vi "Control Loop Process.vi"(8 "error in (no error)":errorcluster, 9 "MainDirectionIn":string, 11 "MPC_Laser Marked in":refnum<class "MPC_Laser Marked.lvclass">) -> (0 "error out":errorcluster, 1 "MainDirectionOut":string, 2 "ProcessAction":string[](array[string]), 3 "MPC_Laser Marked out":refnum<class "MPC_Laser Marked.lvclass">)   [LabVIEW 2019, in "MPC_Laser Marked.lvclass"]
uses:
  MPC_Laser Marked.lvclass
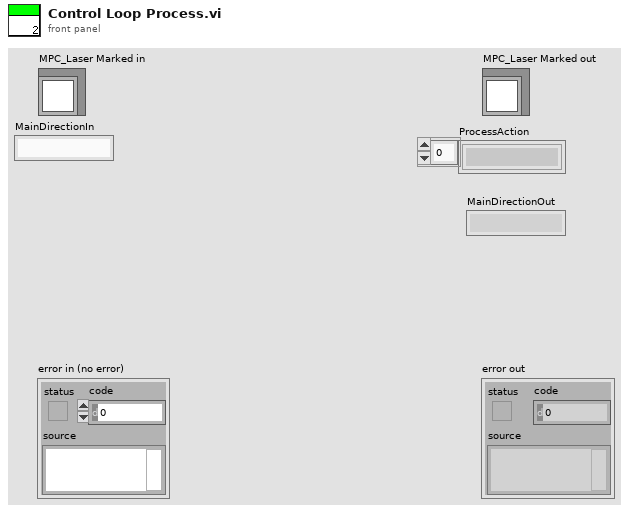
[diagram p1: front panel]
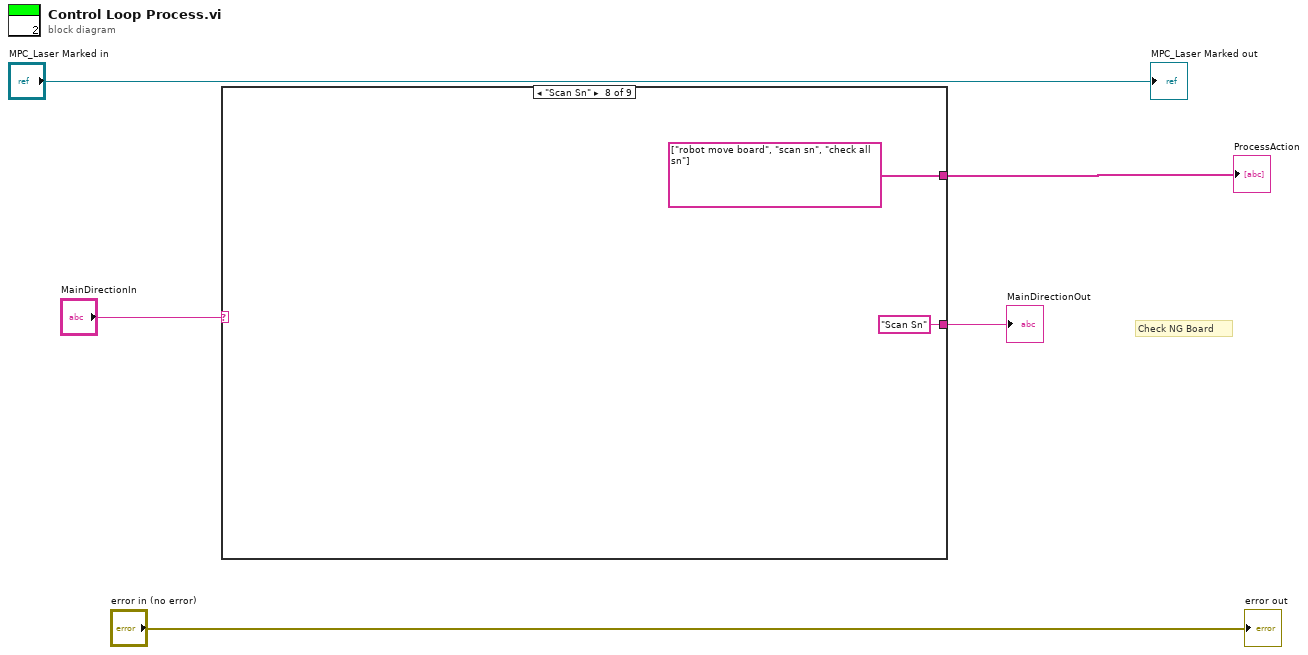
[diagram p0: block diagram]
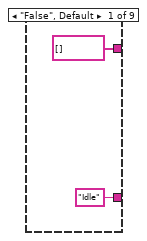
[diagram p2: hidden frame]
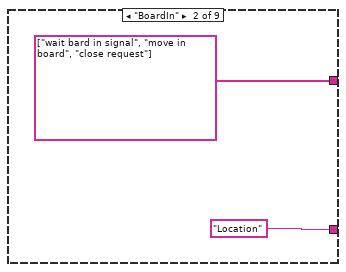
[diagram p3: hidden frame]
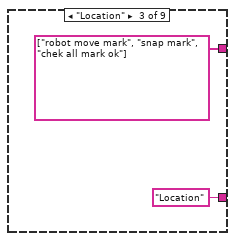
[diagram p4: hidden frame]
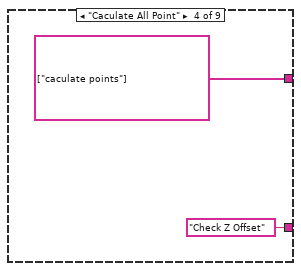
[diagram p5: hidden frame]
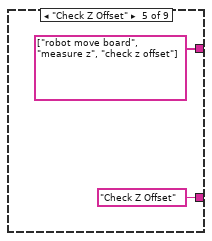
[diagram p6: hidden frame]
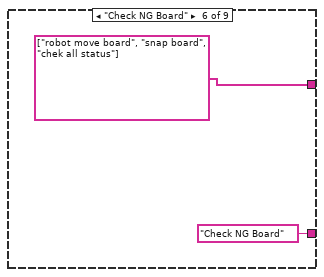
[diagram p7: hidden frame]
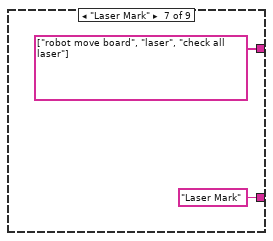
[diagram p8: hidden frame]
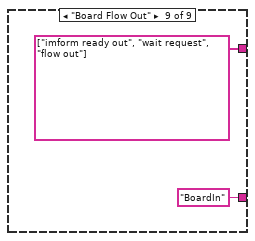
[diagram p9: hidden frame]
diagram:
  # "Check NG Board"
  n1 = case shown="\"Scan Sn\"" "MainDirectionIn" {
    tunnel: [string[] [] string[] ["wait bard in signal", "move in board", "close request"] string[] ["robot move mark", "snap mark", "chek all mark ok"] string[] ["caculate points"] string[] ["robot move board", "measure z", "check z offset"] string[] ["robot move board", "snap board", "chek all status"] string[] ["robot move board", "laser", "check all laser"] string[] ["robot move board", "scan sn", "check all sn"] string[] ["imform ready out", "wait request", "flow out"]] -> w3
    tunnel: ["Idle" "Location" "Location" "Check Z Offset" "Check Z Offset" "Check NG Board" "Laser Mark" "Scan Sn" "BoardIn"] -> w1
    frame "False", Default {
    }
    frame "BoardIn" {
    }
    frame "Location" {
    }
    frame "Caculate All Point" {
    }
    frame "Check Z Offset" {
    }
    frame "Check NG Board" {
    }
    frame "Laser Mark" {
    }
    frame "Scan Sn" {
    }
    frame "Board Flow Out" {
    }
  }
  "ProcessAction" <- w3
  "MainDirectionOut" <- w1
  "error out" <- "error in (no error)"
  "MPC_Laser Marked out" <- "MPC_Laser Marked in"
